vi "test_Add Command_Use SysDef With Only Custom Device.vi"(8 "error in (no error)":errorcluster, 11 "TestCase in":refnum<class "Instrument Addon Scripting API Messages Unit Tests.lvclass">) -> (0 "error out":errorcluster, 3 "TestCase out":refnum<class "Instrument Addon Scripting API Messages Unit Tests.lvclass">)   [LabVIEW 2019, in "Instrument Addon Scripting API Messages Unit Tests.lvclass"]
uses:
  Instrument Addon Scripting API Messages Unit Tests.lvclass
  Addon/Addon Shared/Types/FG Control.ctl
  APIs/Scripting API/TypeDefs/Command Settings.ctl
  <vilib>/NI VeriStand/Custom Device API/Custom Device Item Ref.ctl
  APIs/Scripting API/TypeDefs/Padding.ctl
  Addon/Addon Shared/Types/Command Parameters.ctl
  Addon/Addon Shared/Types/Linked Channel Cluster.ctl
  Instrument Addon Scripting API Messages Unit Tests.lvclass/Instrument Addon Scripting API Messages Unit Tests.ctl
  Addon/Addon Shared/SubVIs/Constants.vi
  <vilib>/NI/NI VeriStand Advanced SysDef API/_SubVIs/SysDef.Search.GUID.vi
  <vilib>/NI VeriStand/Custom Device API/NI VeriStand - Get Item Property.vi
  <vilib>/NI VeriStand/Custom Device API/Get Item Property (String).vi
  <vilib>/NI VeriStand/Custom Device API/Get Item Property (String Array).vi
  <vilib>/NI VeriStand/Custom Device API/Get Item Property (Boolean).vi
  <vilib>/NI VeriStand/Custom Device API/Get Item Property (U32).vi
  <vilib>/NI VeriStand/Custom Device API/NI VeriStand - Set Item Property.vi
  <vilib>/NI VeriStand/Custom Device API/Set Item Property (String).vi
  <vilib>/NI VeriStand/Custom Device API/Set Item Property (String Array).vi
  <vilib>/NI VeriStand/Custom Device API/Set Item Property (Boolean).vi
  <vilib>/NI VeriStand/Custom Device API/Set Item Property (U32).vi
  <vilib>/addons/_JKI Toolkits/VI Tester/TestCase.llb/TestCase.lvclass
  Instrument Addon Scripting API Test Assets/Instrument Addon Scripting API Test Assets.lvclass
  Addon/Addon Shared/Instrument Addon Shared.lvlib
  <vilib>/NI/NI VeriStand Advanced SysDef API/SysDef API/Advanced System Definition.lvlib
  <vilib>/NI VeriStand/Custom Device API/Custom Device API.lvlib
  APIs/Scripting API/Instrument Addon Scripting API.lvlib
  C:/Program Files (x86)/National Instruments/LabVIEW 2019/vi.lib/addons/_JKI Toolkits/VI Tester/TestCase.llb/TestCase.lvclass
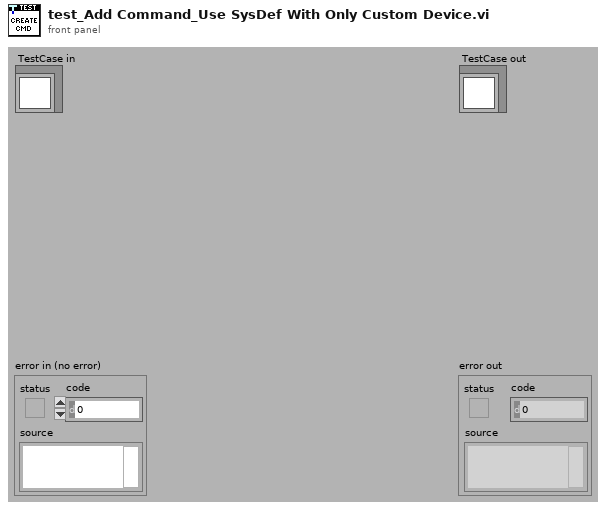
[diagram p1: front panel]
types:
  T1 = typedef "Instrument Addon Scripting API.lvlib/Command Settings.ctl" = cluster{"Command Format":string, "Linked Channels":cluster{"Variable Name":string, "Channel Ref in":T2}[], "Use Padding?":bool, "Padding":T3}
  T2 = typedef "Custom Device API.lvlib/Custom Device Item Ref.ctl" = u64
  T3 = typedef "Instrument Addon Scripting API.lvlib/Padding.ctl" = cluster{"Pad Value":u8, "Length":u32}
  T4 = typedef "Instrument Addon Shared.lvlib/FG Control.ctl" = enum16{"Get", "Set"}
  T5 = typedef "Instrument Addon Shared.lvlib/Command Parameters.ctl" = cluster{"Command":string, "Linked Channels":T6[], "Pad":bool, "Length":u32, "Pad Value":u8}
  T6 = typedef "Instrument Addon Shared.lvlib/Linked Channel Cluster.ctl" = cluster{"Variable Name":string, "GUID":string}
  T7 = typedef "Instrument Addon Scripting API.lvlib/Linked Channel.ctl" = cluster{"Variable Name":string, "Channel Refnum":T2}
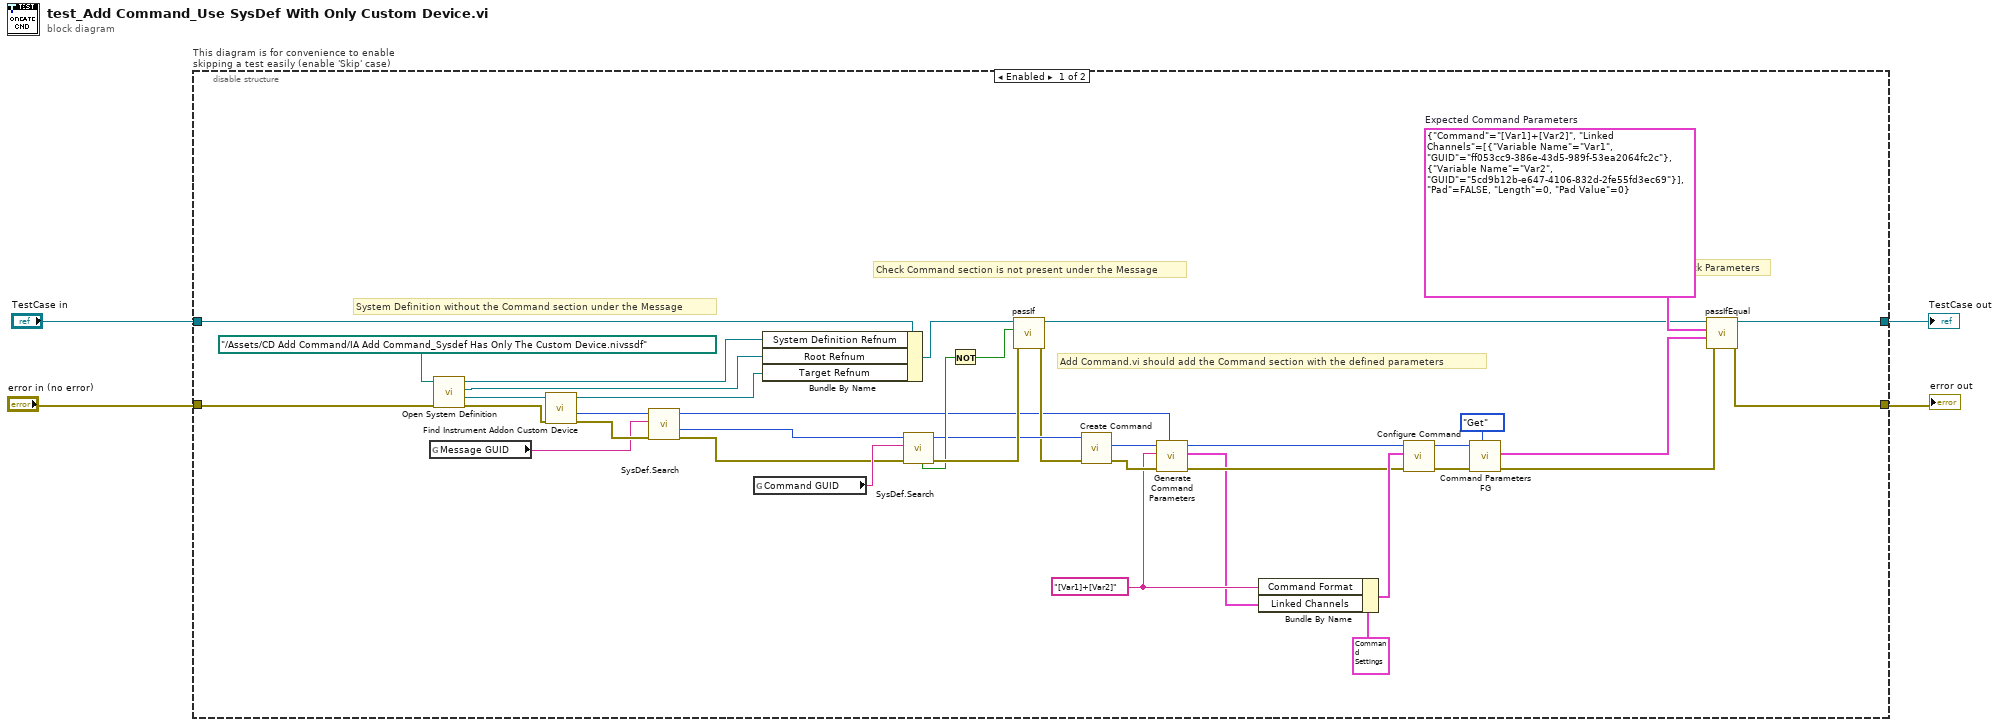
[diagram p0: block diagram]
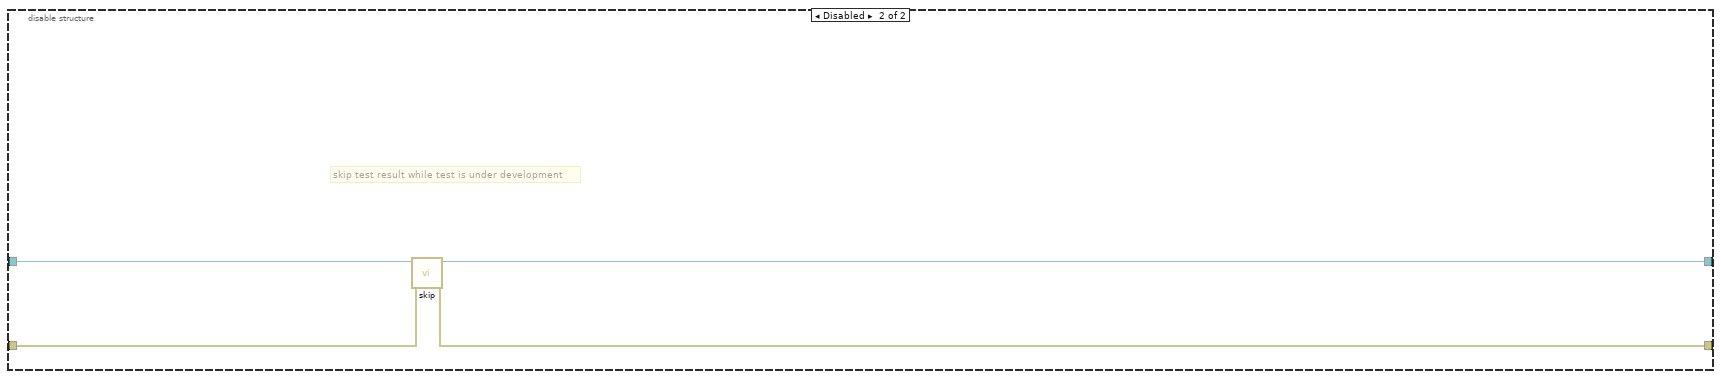
[diagram p2: hidden frame]
diagram:
  n1 = disable-structure "This diagram is for convenience to enable skipping a test easily (enable 'Skip' case)" shown="Enabled" {
    disable-tunnel: "TestCase in" -> [w22 w46]
    disable-tunnel: [w39 w44] -> w1
    disable-tunnel: [w40 w45] -> w3
    disable-tunnel: "error in (no error)" -> [w41 w43]
    frame Enabled {
      w30 = T5 {"Command"="[Var1]+[Var2]", "Linked Channels"=[{"Variable Name"="Var1", "GUID"="ff053cc9-386e-43d5-989f-53ea2064fc2c"}, {"Variable Name"="Var2", "GUID"="5cd9b12b-e647-4106-832d-2fe55fd3ec69"}], "Pad"=FALSE, "Length"=0, "Pad Value"=0}  # Expected Command Parameters
      w7 = "[Var1]+[Var2]" ("Command Format")
      # "Check Command section is not present under the Message"
      # "Add Command.vi should add the Command section with the defined parameters"
      # "System Definition without the Command section under the Message"
      # "Check Parameters"
      n2 = global read "Constants.vi" "Message GUID"() -> (w33:string)
      n3 = call "Open System Definition.vi"("error in (no error)"=w41, "System Definition File"=path "../Assets/CD Add Command/IA Add Command_Sysdef Has Only The Custom Device.nivssdf" ("SDF file")) -> ("error out"=w35:errorcluster, "Target Refnum"=w36:refnum<k24>, "Root Refnum"=w19:refnum<k24>, "System Definition Refnum"=w20:refnum<k24>)  [unwired: 6 in]
      n4 = call "Find Instrument Addon Custom Device.vi"("error in"=w35, "target in"=w36) -> ("error out"=w34:errorcluster, "NodeID"=w31:u64, "target out"=w18:refnum<k24>)  [unwired: 7 in]
      n5 = call-poly <vilib>:"SysDef.Search.vi"("error in (no error)"=w34, "GUID"=w33, "nodeID"=w31) -> ("error out"=w28:errorcluster, "Value out"=w12:u64, "nodeID out"=w5:u64)  [unwired: 5 in, 1 out]
      n6 = global read "Constants.vi" "Command GUID"() -> (w29:string)
      n7 = Bundle By Name(cluster=w22, "System Definition Refnum"=w20, "Root Refnum"=w19, "Target Refnum"=w18) -> (w21:refnum<class "Instrument Addon Scripting API Messages Unit Tests.lvclass">)
      n8 = call-poly <vilib>:"SysDef.Search.vi"("error in (no error)"=w28, "GUID"=w29, "nodeID"=w12) -> ("error out"=w27:errorcluster, "nodeID out"=w14:u64, "Found?"=w25:bool)  [unwired: 5 in, 1 out]
      n9 = Not(x=w25) -> (.not. x?=w24:bool)
      n10 = call-dynamic "passIf.vi"("error in (no error)"=w27, "pass"=w24, "TestCase in"=w21) -> ("error out"=w13:errorcluster, "TestCase out"=w26:refnum<class "Instrument Addon Scripting API Messages Unit Tests.lvclass">)  [unwired: 7 in]
      n11 = call "Create Command.vi"("error in"=w13, "message refnum In"=w14) -> ("error out"=w9:errorcluster, "command refnum"=w11:T2)  [unwired: 7 in, 1 out]
      n12 = call "Generate Command Parameters.vi"("Instrument Addon Refnum in"=w5, "Error In"=w9, "Command String"=w7, "Command Channel in"=w11) -> ("Error Out"=w8:errorcluster, "Linked Channels"=w6:T7[], "Command Channel out"=w10:T2)  [unwired: 4 in, 1 out]
      n13 = Bundle By Name(cluster=T1 {"Command Format"="[Var1]+[Var2]", "Linked Channels"=[{"Variable Name"="Var1", "Channel Ref in"=32}, {"Variable Name"="Var2", "Channel Ref in"=33}], "Use Padding?"=FALSE, "Padding"={"Pad Value"=0, "Length"=0}} ("Settings"), "Command Format"=w7, "Linked Channels"=w6) -> (w17:T1)
      n14 = call "Configure Command.vi"("error in (no error)"=w8, "settings"=w17, "command refnum in"=w10) -> ("error out"=w16:errorcluster, "command refnum out"=w15:T2)  [unwired: 7 in]
      n15 = call "Command Parameters FG.vi"("Action"=FG_Control."Get", "error in (no error)"=w16, "Item Ref in"=w15) -> ("error out"=w38:errorcluster, "Command Parameters"=w37:T5)  [unwired: 6 in, 1 out]
      n16 = call-dynamic "passIfEqual.vi"("error in (no error)"=w38, "y"=w37, "x"=w30, "TestCase in"=w26) -> ("error out"=w40:errorcluster, "TestCase out"=w39:refnum<class "Instrument Addon Scripting API Messages Unit Tests.lvclass">)  [unwired: 6 in]
    }
    frame Disabled {
      # "skip test result while test is under development"
      n17 = call <vilib>:"skip.vi"("error in (no error)"=w43, "TestCase in"=w46) -> ("error out"=w45:errorcluster, "TestCase out"=w44:refnum<class "Instrument Addon Scripting API Messages Unit Tests.lvclass">)  [unwired: 8 in]
    }
  }
  "error out" <- w3
  "TestCase out" <- w1
